vi "Insert Value[] (String[]).vi"(7 "key":string[](array[string]), 8 "error in (no error)":errorcluster, 10 "JSON Data in":string[](array[string]), 11 "JSON Value in":refnum<class "JSON Value.lvclass">) -> (0 "error out":errorcluster, 1 "replaced":bool, 3 "JSON Value out":refnum<class "JSON Value.lvclass">)   [LabVIEW 2016, in "JSON Value.lvclass"]
uses:
  JSON Value.lvclass
  New JSON Value/New JSON (String[]).vi
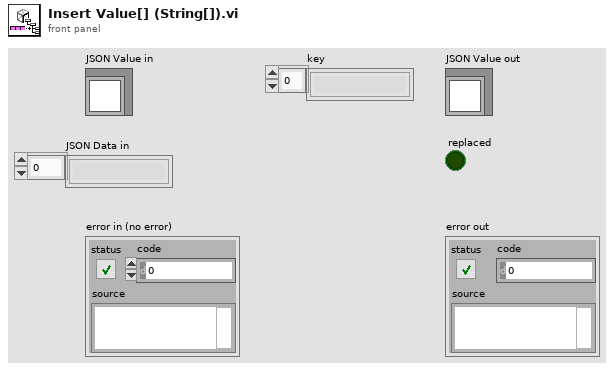
[diagram p1: front panel]
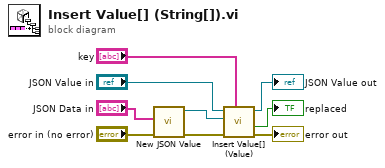
[diagram p0: block diagram]
diagram:
  n1 = call-poly "New JSON Value.vi"("error in (no error)"="error in (no error)", "String Array"="JSON Data in") -> ("error out"=w8:errorcluster, "JSON Value out"=w9:refnum<class "JSON Value.lvclass">)  [unwired: 8 in]
  n2 = call "Insert Value[] (Value).vi"("key"="key", "error in (no error)"=w8, 10:"JSON Value in"=w9, 11:"JSON Value in"="JSON Value in") -> ("error out"=→"error out":errorcluster, "replaced"=→"replaced":bool, "JSON Value out"=→"JSON Value out":refnum<class "JSON Value.lvclass">)  [unwired: 5 in]
